vi "PID Simulation.vi"() -> ()   [LabVIEW 2019]
panel:
  in  "Setpoint 2":dbl(slide)=2.585034013605444 scale=-20.0..20.0
  in  "Profiled?":bool=TRUE
  in  "PIDF Gains":cluster{"Kp":dbl, "Ki":dbl, "Kd":dbl, "Kf":dbl}={"Kp"=5.0, "Ki"=0.0, "Kd"=2.0, "Kf"=0.0} {"Kf" format="%.3f"; "Kd" format="%.3f"; "Ki" format="%.3f"; "Kp" format="%.3f"}
  in  "Output Range":cluster{"output high":dbl, "output low":dbl}={"output high"=1.0, "output low"=-1.0}
  in  "Contraints":T1={"Max Velocity"=2.0, "Max Acceleration"=5.0}
  in  "Config":T2={"Gear Reduction"=15.0, "Wheel Radius (m)"=0.076, "# Motors"=1, "coeff of friction"=0.1, "Mass (kg)"=50.0, "Motor"={"Ke (V)"=0.0183, "R (ohms)"=0.09, "KT (Nm/A)"=0.0183, "Tf (Nm)"=0.4}}
  out "Waveform Chart":T3(graph)={"Position"=2.5841635372992755, "Velocity"=0.09329931972789356, "Velocity"=2.0136243047022866e-11, "Position"=2.5638138105148074, "output"=0.10174863387979682}
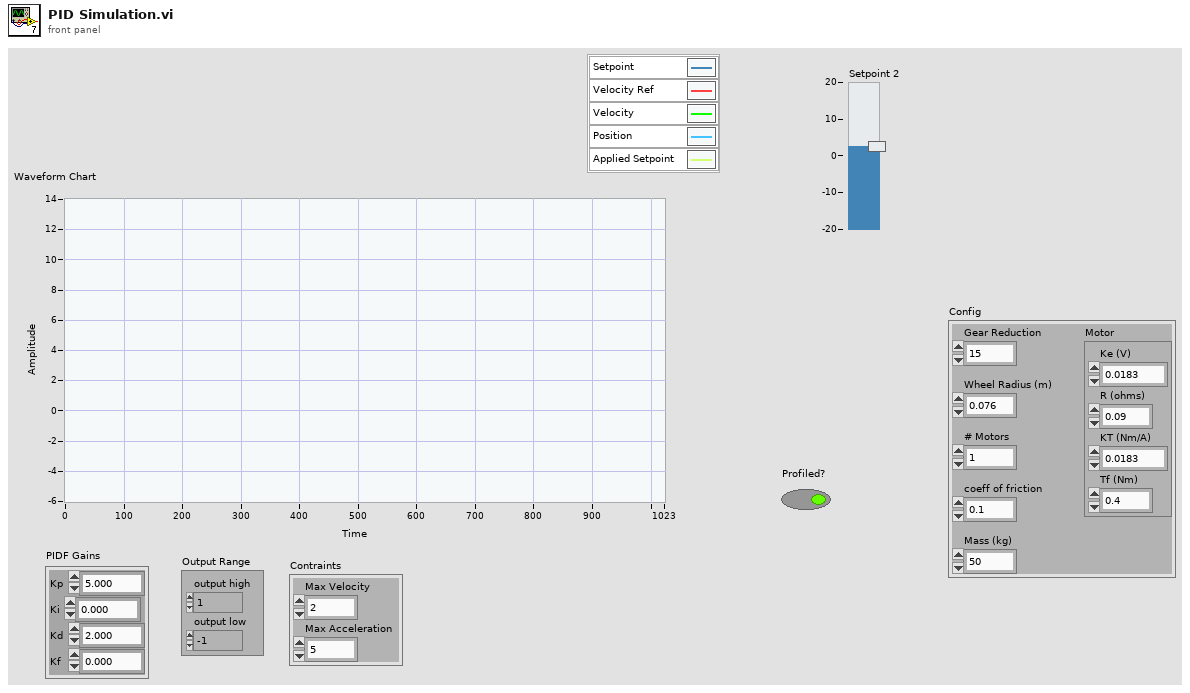
[diagram p1: front panel]
types:
  T1 = cluster{"Max Velocity":dbl, "Max Acceleration":dbl}
  T2 = cluster{"Gear Reduction":dbl, "Wheel Radius (m)":dbl, "# Motors":u32, "coeff of friction":dbl, "Mass (kg)":dbl, "Motor":cluster{"Ke (V)":dbl, "R (ohms)":dbl, "KT (Nm/A)":dbl, "Tf (Nm)":dbl}}
  T3 = cluster{"Position":dbl, "Velocity":dbl, "Velocity":dbl, "Position":dbl, "output":dbl}
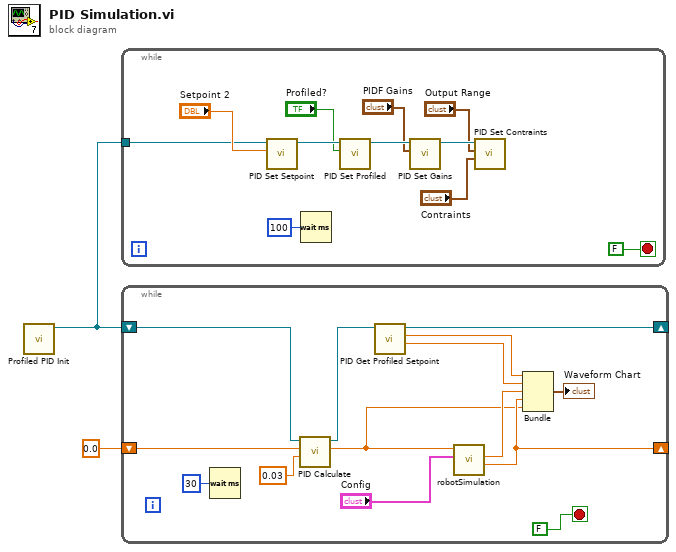
[diagram p0: block diagram]
diagram:
  n1 = call "Profiled PID Init.vi"() -> ("PID Ref"=w1:refnum<data-value>)  [unwired: 11 in]
  n2 = while {
    tunnel: w1 -> [w11]
    stop <- FALSE stop-if-true
    n3 = call "PID Set Setpoint.vi"("Setpoint"="Setpoint 2", "PID Ref"=w11) -> ("PID Ref"=w9:refnum<data-value>)  [unwired: 9 in]
    n4 = Wait (ms)(milliseconds to wait=u32 100) -> ()  [unwired: 1 out]
    n5 = call "PID Set Profiled.vi"("Profiled?"="Profiled?", "PID Ref"=w9) -> ("PID Ref"=w7:refnum<data-value>)  [unwired: 9 in]
    n6 = call "PID Set Gains.vi"("PIDF Gains"="PIDF Gains", "PID Ref"=w7) -> ("PID Ref"=w6:refnum<data-value>)  [unwired: 9 in]
    n7 = call "PID Set Contraints.vi"("Profiled Contraints"="Contraints", "Output Range"="Output Range", "PID Ref"=w6) -> ()  [unwired: 8 in, 1 out]
  }
  n8 = while {
    shift-right: [w24] -> _
    shift-left: 0.0 ("Plant Output") -> [w22]
    shift-right: [w14] -> _
    shift-left: w1 -> [w20]
    stop <- FALSE ("stop") stop-if-true
    n9 = Wait (ms)(milliseconds to wait=u32 30) -> ()  [unwired: 1 out]
    n10 = call "PID Calculate.vi"("dt (s)"=0.03, "Process Variable"=w22, "PID Ref in"=w20) -> ("output"=w16:dbl, "PID Ref out"=w15:refnum<data-value>)  [unwired: 7 in]
    n11 = call "PID Get Profiled Setpoint.vi"("Data Value Reference in"=w15) -> ("Velocity"=w18:dbl, "Position"=w19:dbl, "Data Value Reference out"=w14:refnum<data-value>)  [unwired: 8 in]
    n12 = call "robotSimulation.vi"("Config"="Config", "Duty Cycle"=w16) -> ("Position"=w24:dbl, "Velocity"=w25:dbl)  [unwired: 7 in, 1 out]
    n13 = Bundle("Position"=w19, "Velocity"=w18, "Velocity"=w25, "Position"=w24, "output"=w16) -> (→"Waveform Chart":T3)  [unwired: 1 in]
  }
